vi "ReadFiles.vi"(8 "error in (no error)":errorcluster, 11 "Master in":refnum<class "Master.lvclass">) -> (0 "error out":errorcluster, 3 "Master out":refnum<class "Master.lvclass">)   [LabVIEW 2014, in "Master.lvclass"]
uses:
  Master/Master.lvclass
  Master/Master.lvclass/Master.ctl
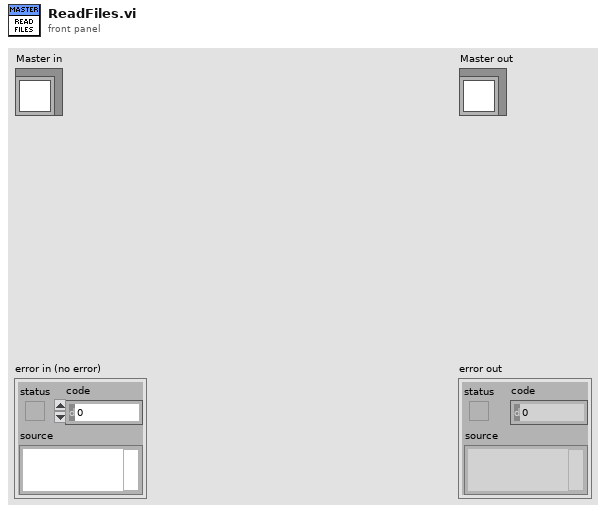
[diagram p1: front panel]
types:
  T1 = enum16{"open", "replace", "create", "open or create", "replace or create", "replace or create with confirmation"}
  T2 = cluster{"type string":i16[], "data string":string}
  T3 = cluster{"type string":i16[], "data string":string}[]
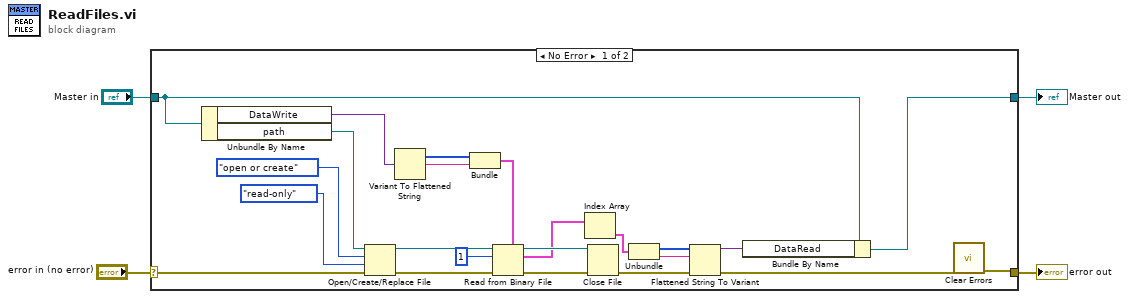
[diagram p0: block diagram]
diagram:
  n1 = case shown="No Error" "error in (no error)" {
    selector: "error in (no error)" -> [w24 w29]
    tunnel: [w5 w29] -> w3
    tunnel: [w14 w28] -> w1
    tunnel: "Master in" -> [w15 w28]
    frame No Error {
      n2 = Unbundle By Name(w15) -> ("DataWrite"=w9:variant, "path"=w27:path)
      n3 = Open/Create/Replace File(file path (use dialog)=w27, error in=w24, operation (0:open)=T1."open or create", access (0:read/write)=enum16{"read/write", "read-only", "write-only"}."read-only") -> (refnum out=w23:refnum<file>, error out=w22:errorcluster)  [unwired: 2 in, 1 out]
      n4 = Variant To Flattened String(Variant=w9) -> (data string=w11:string, 1:w8:i16[])
      n5 = Bundle("type string"=w8, "data string"=w11) -> (w10:T2)  [unwired: 1 in]
      n6 = Read from Binary File(5:w10, 8:w22, 10:1 ("count (1)"), 11:w23) -> (0:w20:errorcluster, 2:w19:T3, 3:w21:refnum<file>)  [unwired: 2 in, 1 out]
      n7 = Index Array(array=w19) -> (element=w18:T2)  [unwired: 1 in]
      n8 = Close File(refnum=w21, error in=w20) -> (error out=w16:errorcluster)  [unwired: 1 out]
      n9 = Unbundle(w18) -> ("type string"=w17:i16[], "data string"=w7:string)
      n10 = Flattened String To Variant(4:w16, 6:w7, 7:w17) -> (0:w6:errorcluster, 3:w13:variant)
      n11 = Bundle By Name(cluster=w15, "DataRead"=w13) -> (w14:refnum<class "Master.lvclass">)
      n12 = call <vilib>:"Clear Errors.vi"("error in (no error)"=w6) -> ("error out"=w5:errorcluster)  [unwired: 5 in, 1 out]
    }
    frame Error {
    }
  }
  "error out" <- w3
  "Master out" <- w1
